vi "Create Sessions Dispatcher.vi"(7 "require single session":bool, 8 "error in":errorcluster, 10 "instrument":refnum<class "IInstrument.lvclass">, 11 "session reservation in":refnum<class "Session Reservation.lvclass">) -> (0 "error out":errorcluster, 1 "channel lists":string[](array[string]), 2 "sessions":variant[](array[variant]), 3 "session reservation out":refnum<class "Session Reservation.lvclass">)   [LabVIEW 2020, in "MeasurementLink Session Management.lvlib" / "Session Reservation.lvclass"]
uses:
  Session Reservation.lvclass
  MeasurementLink Instrument/IInstrument/IInstrument.lvclass
  Session Reservation.lvclass/Session Reservation.ctl
  IState/IState.lvclass
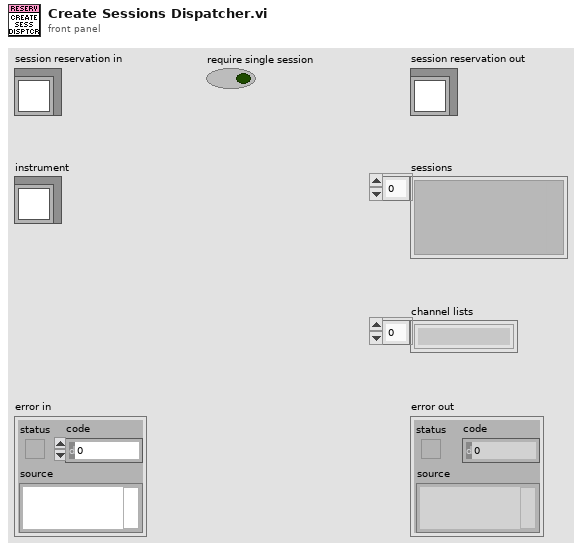
[diagram p1: front panel]
types:
  T1 = typedef "MeasurementLink Session Management.lvlib/Session Reservation.lvclass/Data.ctl" = cluster{"session and driver infos":T2[], "pin or relay names":string[], "connection map":refnum<class "Connection Map.lvclass">, "pin map context":T6, "state":refnum<class "IState.lvclass">}
  T2 = typedef "MeasurementLink Session Management.lvlib/Session Reservation.lvclass/Session and Driver Info.ctl" = cluster{"session info":T3, "session":variant, "instrument":refnum<class "IInstrument.lvclass">}
  T3 = typedef "MeasurementLink Session Management Client.lvlib/ni_measurementlink_sessionmanagement_v1_SessionInformation.ctl" = cluster{"session":T4, "resource_name":string, "channel_list":string, "instrument_type_id":string, "session_exists":bool, "channel_mappings":T5[]}
  T4 = typedef "MeasurementLink Session Management Client.lvlib/nidevice_grpc_Session.ctl" = cluster{"name":string}
  T5 = typedef "MeasurementLink Session Management Client.lvlib/ni_measurementlink_sessionmanagement_v1_ChannelMapping.ctl" = cluster{"pin_or_relay_name":string, "site":i32, "channel":string}
  T6 = typedef "MeasurementLink Session Management Client.lvlib/ni_measurementlink_PinMapContext.ctl" = cluster{"pin_map_id":string, "sites":i32[]}
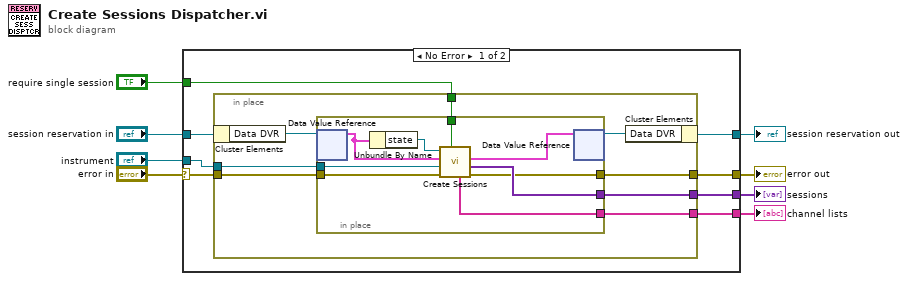
[diagram p0: block diagram]
diagram:
  n1 = case shown="No Error" "error in" {
    selector: "error in" -> [w15 w35]
    tunnel: [w14 w35] -> w7
    tunnel: [w10 w34] -> w5
    tunnel: "session reservation in" -> [w16 w34]
    tunnel: "require single session" -> [w13 _]
    tunnel: "instrument" -> [w12 _]
    tunnel: [w11 _] -> w2
    tunnel: [w9 _] -> w1
    frame No Error {
      n2 = in-place {
        in-place-border: w15 -> [w23]
        in-place-border: [w22] -> w14
        in-place-border: w13 -> [w21]
        in-place-border: w12 -> [w20]
        in-place-border: [w19] -> w11
        in-place-border: [w17] -> w9
        n3 = in-place-cluster #1(w16) -> ("Data DVR"=w24:refnum<data-value>)
        n4 = in-place {
          in-place-border: w23 -> [w29]
          in-place-border: [w26] -> w22
          in-place-border: w21 -> [w31]
          in-place-border: w20 -> [w28]
          in-place-border: [w25] -> w19
          in-place-border: [w27] -> w17
          n5 = in-place-dvr #2(w24) -> (w30:T1)  [unwired: 1 out]
          n6 = Unbundle By Name(w30) -> ("state"=w33:refnum<class "IState.lvclass">)
          n7 = call-dynamic "Create Sessions.vi"("require single session"=w31, "error in"=w29, "instrument"=w28, "data in"=w30, "state in"=w33) -> ("error out"=w26:errorcluster, "sessions"=w27:variant[], "data out"=w32:T1, "channel lists"=w25:string[])  [unwired: 3 in]
          n8 = in-place-dvr #2(w32) -> (w18:refnum<data-value>)  [unwired: 1 out]
        }
        n9 = in-place-cluster #1("Data DVR"=w18) -> (w10:refnum<class "Session Reservation.lvclass">)
      }
    }
    frame Error {
    }
  }
  "error out" <- w7
  "session reservation out" <- w5
  "sessions" <- w1
  "channel lists" <- w2
